vi "Mouse Down.vi"(8 "error in (no error)":errorcluster, 10 "Cell Position":T1, 11 "MCLB_Template in":refnum<class "MCLB_Template.lvclass">) -> (0 "error out":errorcluster, 3 "MCLB_Template out":refnum<class "MCLB_Template.lvclass">)   [LabVIEW 2021, in "MCLB_Template.lvclass"]
uses:
  MCLB_Template.lvclass
  <vilib>/Utility/miscctls.llb/LVRowAndColumnTypeDef.ctl
  MCLB_Template.lvclass/MCLB_Template.ctl
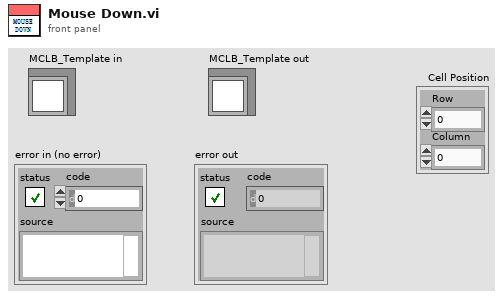
[diagram p1: front panel]
types:
  T1 = typedef "LVRowAndColumnTypeDef.ctl" = cluster{"Row":i32, "Column":i32}
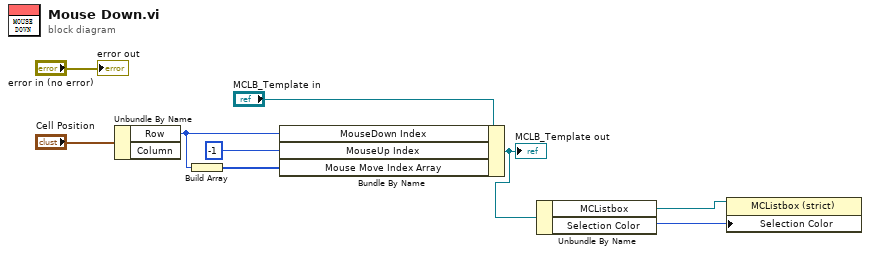
[diagram p0: block diagram]
diagram:
  n1 = Unbundle By Name("Cell Position") -> ("Row"=w7:i32)  [unwired: 1 out]
  n2 = Build Array(w7) -> (w5:i32[])
  n3 = Bundle By Name(cluster="MCLB_Template in", "MouseDown Index"=w7, "MouseUp Index"=-1 ("MouseSelect.MouseUp Index"), "Mouse Move Index Array"=w5) -> (w3:refnum<class "MCLB_Template.lvclass">)
  "MCLB_Template out" <- w3
  n4 = Unbundle By Name(w3) -> ("MCListbox"=w2:refnum<vi>, "Selection Color"=w1:u32)
  n5 = property on="Property Node" class="MCListbox (strict)"(reference=w2, "Selection Color"=w1) -> ()  [unwired: 1 in, 2 out]
  "error out" <- "error in (no error)"
